vi "update accessory panels.vi"(5 "tracking":bool, 6 "spilt ff/fb":bool, 7 "xyz order":bool, 8 "error in (no error)":errorcluster, 9 "scaling info":T2={" scan settings"={"z resolution (pixels)"=0, "iterations per pixel"=0, "iterations per z-scan (=zres*iterperpixel)"=0, "x resolution (pixels)"=0, "y resolution (pixels)"=0, "number of z-lines per volume"=0, "number of repetitions (volumes)"=0, "Pockels cell voltage (bits)"=0, "Vx center (bits)"=0, "Vy center (bits)"=0, "Vx amplitude (bits)"=0, "Vy amplitude (bits)"=0, "lines to delay between scan start and output"=0, "LSB has acquire control"=FALSE, "Pockels cell bleach voltage"=0}, "scale factors (um/level)"=[0.016, 0.016, 0.00025], "z-feedback range"=2560, "r sphere/sigma"=180.0}, 10 "stop":bool, 11 "refs":T4) -> (0 "error out":errorcluster, 2 "location constraints":T3(array[cluster]), 4 "num spots":u8)   [LabVIEW 2010]
uses:
  scan_specification_tagResonant.ctl
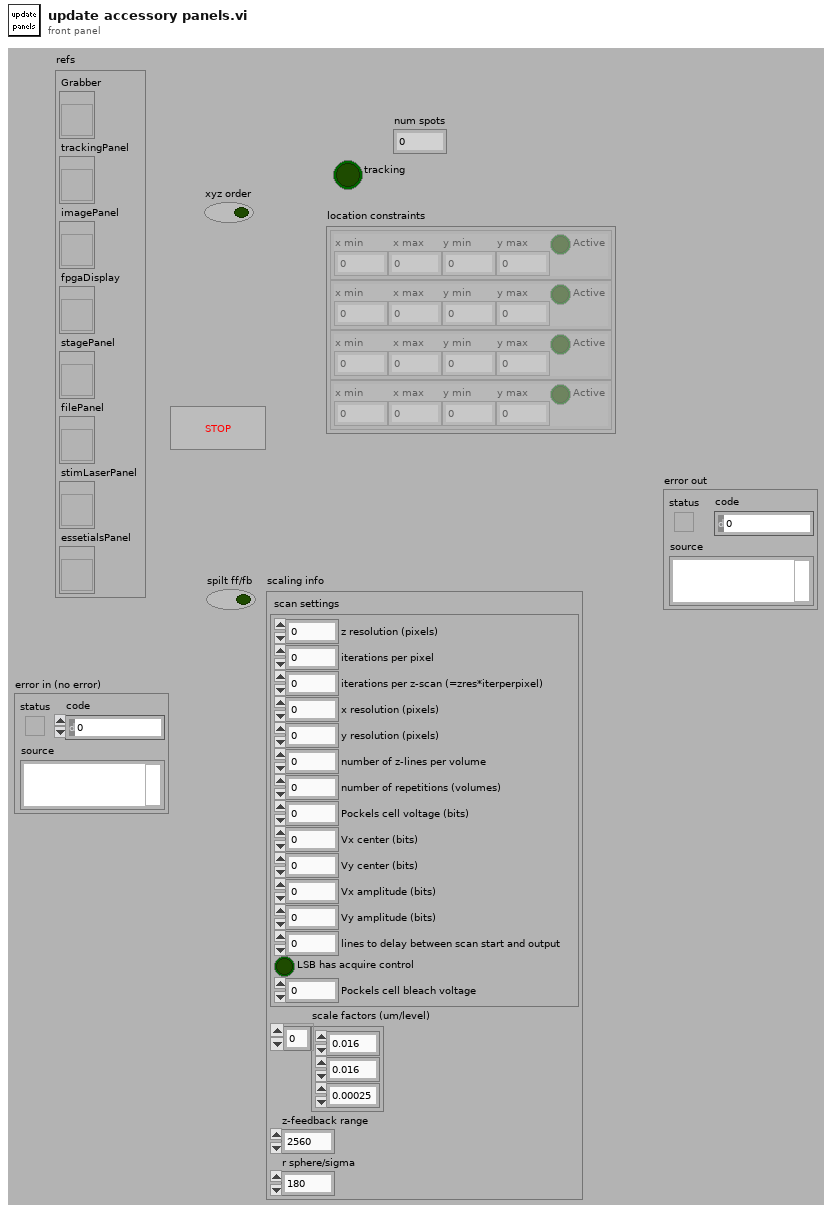
[diagram p1: front panel]
types:
  T1 = typedef "scan_specification_tagResonant.ctl" = cluster{"z resolution (pixels)":u16, "iterations per pixel":u16, "iterations per z-scan (=zres*iterperpixel)":u16, "x resolution (pixels)":u16, "y resolution (pixels)":u16, "number of z-lines per volume":u16, "number of repetitions (volumes)":i32, "Pockels cell voltage (bits)":i16, "Vx center (bits)":i16, "Vy center (bits)":i16, "Vx amplitude (bits)":i16, "Vy amplitude (bits)":i16, "lines to delay between scan start and output":u16, "LSB has acquire control":bool, "Pockels cell bleach voltage":i16}
  T2 = cluster{" scan settings":T1, "scale factors (um/level)":dbl[], "z-feedback range":i16, "r sphere/sigma":dbl}
  T3 = cluster{"x min":i32, "x max":i32, "y min":i32, "y max":i32, "Active":bool}[]
  T4 = cluster{"Grabber":refnum<vi>, "trackingPanel":refnum<vi>, "imagePanel":refnum<vi>, "fpgaDisplay":refnum<vi>, "stagePanel":refnum<vi>, "filePanel":refnum<vi>, "stimLaserPanel":refnum<vi>, "essetialsPanel":refnum<vi>}
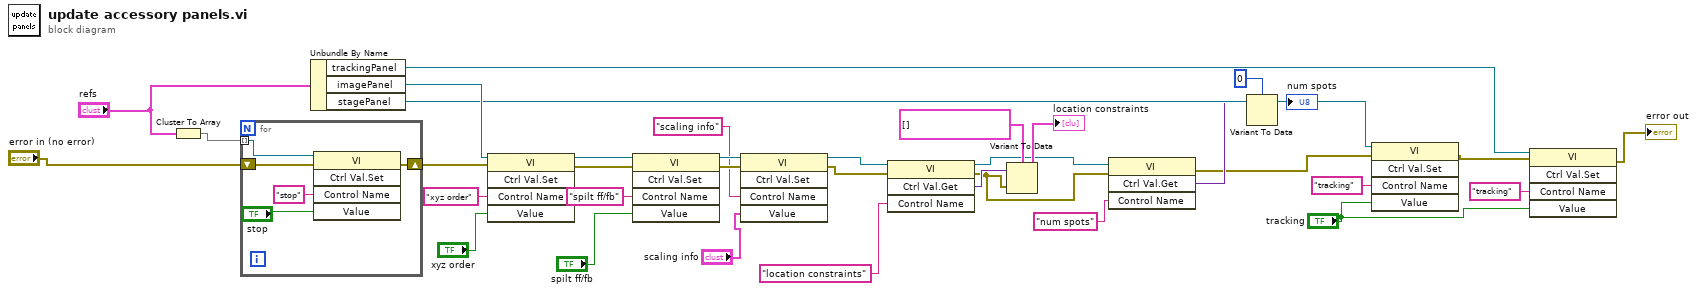
[diagram p0: block diagram]
diagram:
  n1 = Cluster To Array(cluster="refs") -> (array=w33:refnum<vi>[])
  n2 = for {
    tunnel: w33 -> [w37] mode=indexing
    shift-right: [w36] -> w32
    shift-left: "error in (no error)" -> [w40]
    n3 = invoke class="VI" method="Ctrl Val.Set"(reference=w37, error in=w40, "Control Name"="stop", "Value"="stop") -> (error out=w36:errorcluster)  [unwired: 1 in, 4 out]
  }
  n4 = Unbundle By Name("refs") -> ("trackingPanel"=w16:refnum<vi>, "imagePanel"=w31:refnum<vi>, "stagePanel"=w21:refnum<vi>)
  n5 = invoke class="VI" method="Ctrl Val.Set"(reference=w31, error in=w32, "Control Name"="xyz order", "Value"="xyz order") -> (reference out=w28:refnum<vi>, error out=w27:errorcluster)  [unwired: 1 in, 3 out]
  n6 = invoke class="VI" method="Ctrl Val.Set"(reference=w28, error in=w27, "Control Name"="spilt ff/fb", "Value"="spilt ff/fb") -> (reference out=w23:refnum<vi>, error out=w24:errorcluster)  [unwired: 1 in, 3 out]
  n7 = invoke class="VI" method="Ctrl Val.Set"(reference=w23, error in=w24, "Control Name"="scaling info", "Value"="scaling info") -> (reference out=w7:refnum<vi>, error out=w6:errorcluster)  [unwired: 1 in, 3 out]
  n8 = invoke class="VI" method="Ctrl Val.Get"(reference=w7, error in=w6, "Control Name"="location constraints") -> (reference out=w3:refnum<vi>, error out=w2:errorcluster, "Get Control Value Variant"=w14:variant)  [unwired: 1 in, 1 out]
  n9 = Variant To Data(error in=w2, Variant=w14, type=T3 [] ("location constraints")) -> (data=→"location constraints":T3)  [unwired: 1 out]
  n10 = invoke class="VI" method="Ctrl Val.Get"(reference=w3, error in=w2, "Control Name"="num spots") -> (error out=w8:errorcluster, "Get Control Value Variant"=w11:variant)  [unwired: 1 in, 2 out]
  n11 = Variant To Data(Variant=w11, type=u8 0) -> (data=→"num spots":u8)  [unwired: 1 in, 1 out]
  n12 = invoke class="VI" method="Ctrl Val.Set"(reference=w21, error in=w8, "Control Name"="tracking", "Value"="tracking") -> (error out=w18:errorcluster)  [unwired: 1 in, 4 out]
  n13 = invoke class="VI" method="Ctrl Val.Set"(reference=w16, error in=w18, "Control Name"="tracking", "Value"="tracking") -> (error out=→"error out":errorcluster)  [unwired: 1 in, 4 out]
